vi "gen_pulse_train.vi"(7 "sampling rate":dbl format="%#_6p", 9 "waiting time":dbl format="%#_6p", 10 "pulse width":dbl format="%#_6p", 11 "Number of pulses":i32) -> (0 "waveform length":i32, 3 "digital waveform out":digitalwaveform(waveform)={"t0"=timestamp(0 s since 1904-01-01), "dt"=0.0, "Y"={"transitions"=[], "data"=[]}, "error"={"status"=FALSE, "code"=37421928, "source"=""}})   [LabVIEW 2019]
uses:
  <vilib>/Waveform/WDTOps.llb/WDT Scale Delta t DBL.vi
  <vilib>/Waveform/WDTOps.llb/WDT Append Waveforms DBL.vi
  <vilib>/Waveform/DWDTOps.llb/DWDT Analog to Digital.vi
  <vilib>/Waveform/DWDTOps.llb/DWDT Digital to Analog.vi
  <vilib>/Waveform/WDTOps.llb/WDT Number of Waveform Samples DBL.vi
  <vilib>/measure/NI_MABase.lvlib
panel:
  out "Reconverted Pulse train":waveform(dbl)(graph)
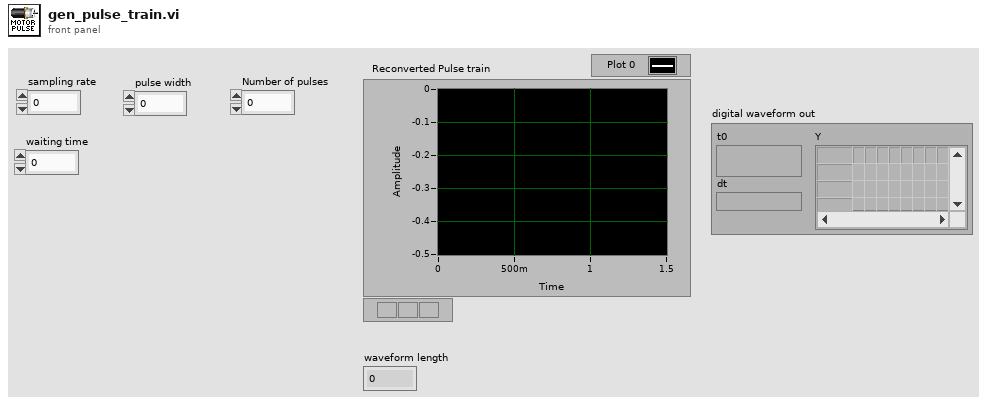
[diagram p1: front panel]
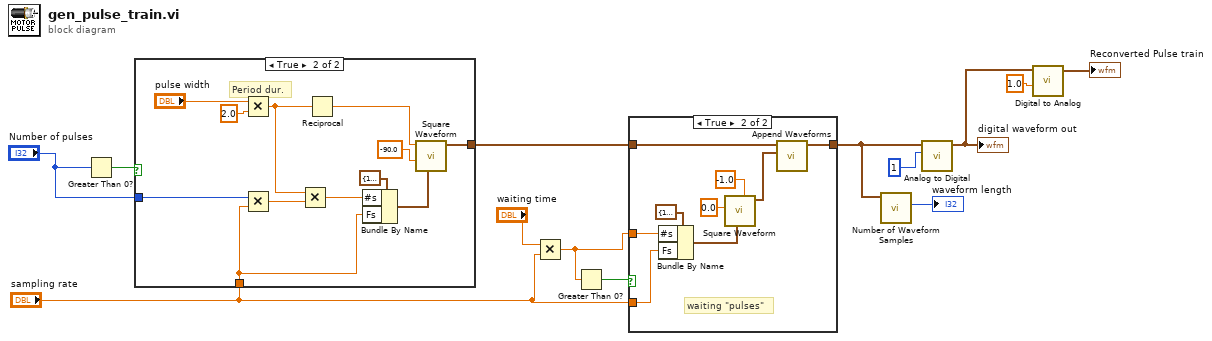
[diagram p0: block diagram]
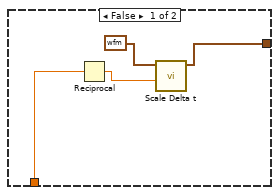
[diagram p2: hidden frame]
diagram:
  n1 = Greater Than 0?(x="Number of pulses") -> (x > 0?=w3:bool)
  n2 = case shown="True" w3 {
    tunnel: [w14 w21] -> w9
    tunnel: "sampling rate" -> [w16 w19]
    tunnel: "Number of pulses" -> [_ w18]
    frame False {
      n3 = Reciprocal(x=w16) -> (1/x=w17:dbl)
      n4 = call-poly <vilib>:"Scale Delta t.vi"("scale factor"=w17, "waveform in"=waveform(dbl) {"t0"=timestamp(0 s since 1904-01-01), "dt"=1.0, "Y"=[]} ("Waveform")) -> ("waveform out"=w14:waveform(dbl))  [unwired: 8 in, 1 out]
    }
    frame True {
      # "Period dur."
      n5 = Multiply(x="pulse width", y=2.0) -> (x*y=w22:dbl)
      n6 = Multiply(x=w18, y=w19) -> (x*y=w23:dbl)
      n7 = Multiply(x=w22, y=w23) -> (x*y=w20:dbl)
      n8 = Reciprocal(x=w22) -> (1/x=w24:dbl)
      n9 = Bundle By Name(cluster=cluster{"Fs":dbl, "#s":dbl} {"Fs"=1000.0, "#s"=1000.0} ("sampling info"), "#s"=w20, "Fs"=w19) -> (w25:cluster{"Fs":dbl, "#s":dbl})
      n10 = call <vilib>:"Square Waveform.vi"("sampling info"=w25, "phase"=-90.0, "frequency"=w24) -> ("signal out"=w21:waveform(dbl))  [unwired: 7 in, 1 out]
    }
  }
  n11 = Multiply(x="waiting time", y="sampling rate") -> (x*y=w6:dbl)
  n12 = Greater Than 0?(x=w6) -> (x > 0?=w5:bool)
  n13 = case shown="True" w5 {
    tunnel: w6 -> [_ w35]
    tunnel: w9 -> [w30 w34]
    tunnel: "sampling rate" -> [_ w31]
    tunnel: [w30 w32] -> w8
    frame False {
    }
    frame True {
      # "waiting \"pulses\""
      n14 = Bundle By Name(cluster=cluster{"Fs":dbl, "#s":dbl} {"Fs"=1000.0, "#s"=1000.0} ("sampling info"), "#s"=w35, "Fs"=w31) -> (w36:cluster{"Fs":dbl, "#s":dbl})
      n15 = call <vilib>:"Square Waveform.vi"("offset"=-1.0, "sampling info"=w36, "amplitude"=0.0) -> ("signal out"=w33:waveform(dbl))  [unwired: 7 in, 1 out]
      n16 = call-poly <vilib>:"Append Waveforms.vi"("waveform B"=w33, "waveform A"=w34) -> ("waveform out"=w32:waveform(dbl))  [unwired: 8 in, 1 out]
    }
  }
  n17 = call-poly <vilib>:"Number of Waveform Samples.vi"("waveform in"=w8) -> ("number of samples"=→"waveform length":i32)  [unwired: 8 in, 2 out]
  n18 = call-poly <vilib>:"Analog to Digital.vi"("resolution (16 bit)"=1, "analog waveform"=w8) -> ("digital waveform"=w12:digitalwaveform)  [unwired: 6 in, 3 out]
  "digital waveform out" <- w12
  n19 = call-poly <vilib>:"Digital to Analog.vi"("full-scale range (pk-pk)"=1.0, "digital waveform"=w12) -> ("analog waveform"=→"Reconverted Pulse train":waveform(dbl))  [unwired: 6 in, 3 out]
